vi "Update.vi"(7 "Parent ID":string, 8 "Error In":errorcluster, 10 "Option String":string, 11 "Tree Manager":T1) -> (0 "Error Out":errorcluster, 3 "Tree Manager":T1)   [LabVIEW 2020, in "NI_VIAnCFGDataStructure.lvlib" / "Tree.lvclass"]
doc: "Call the Update method defined for all the Tree Data types stored as the arguments of the specified Tree. If you prefer to call the Update on a specific argument only Get, Update and Set the argument using basic Tree API calls.\n\nTo define new functionality for Update create child classes of Tree Data.lvclass and override the behavior of the parent for Update method."
uses:
  <vilib>/addons/analyzer/VIAnCFGDataStructure/Tree Manager/Tree.lvclass
  <vilib>/addons/analyzer/VIAnCFGDataStructure/Tree Manager/Typedefs/Session Handle.ctl
  <vilib>/addons/analyzer/VIAnCFGDataStructure/Tree Manager/Tree.lvclass/Tree.ctl
  <vilib>/addons/analyzer/VIAnCFGDataStructure/Tree Data/Tree Data.lvclass
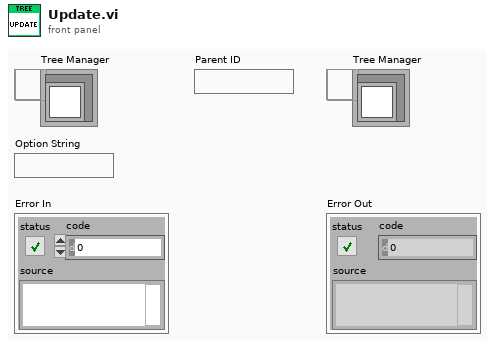
[diagram p1: front panel]
types:
  T1 = typedef "NI_VIAnCFGDataStructure.lvlib/Tree.lvclass/Session Handle.ctl" = refnum<data-value>
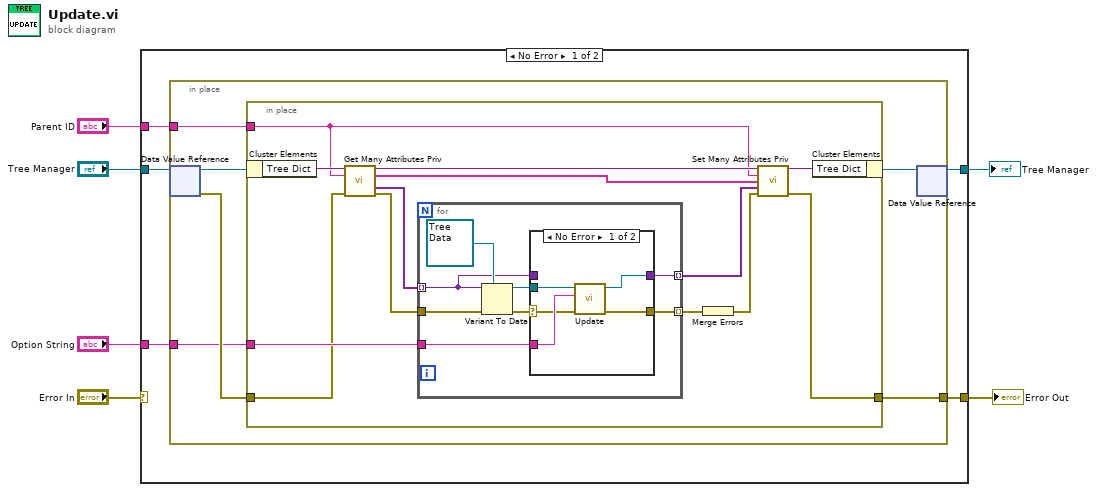
[diagram p0: block diagram]
diagram:
  n1 = case shown="No Error" "Error In" {
    selector: "Error In" -> [_ w45]
    tunnel: "Tree Manager" -> [w11 w46]
    tunnel: [w10 w46] -> w5
    tunnel: [w9 w45] -> w3
    tunnel: "Parent ID" -> [w8 _]
    tunnel: "Option String" -> [w7 _]
    frame No Error {
      n2 = in-place {
        in-place-border: [w16] -> w9
        in-place-border: w8 -> [w13]
        in-place-border: w7 -> [w12]
        n3 = in-place-dvr #1(w11) -> (w17:refnum<class "Tree.lvclass">, w14:errorcluster)
        n4 = in-place {
          in-place-border: [w19] -> w16
          in-place-border: w14 -> [w22]
          in-place-border: w13 -> [w20]
          in-place-border: w12 -> [w26]
          n5 = in-place-cluster #2(w17) -> ("Tree Dict"=w30:variant)
          n6 = call <vilib>:"Get Many Attributes Priv.vi"("Tree Dictionary In"=w30, "Unique ID"=w20, "error in"=w22) -> ("Tree Dictionary Out"=w29:variant, "Attribute Names"=w18:string[], "Attribute Values"=w27:variant[], "error out"=w23:errorcluster)  [unwired: 8 in, 1 out]
          n7 = for {
            tunnel: w27 -> [w33] mode=indexing
            tunnel: w26 -> [w35]
            tunnel: [w34] -> w25 mode=indexing
            tunnel: [w32] -> w24 mode=indexing
            tunnel: w23 -> [w31]
            n8 = Variant To Data(error in=w31, type=refnum<class "Tree Data.lvclass"> refnum ("Tree Data.lvclass"), Variant=w33) -> (data=w36:refnum<class "Tree Data.lvclass">, error out=w37:errorcluster)
            n9 = case shown="No Error" w37 {
              selector: w37 -> [w41 _]
              tunnel: w36 -> [w43 _]
              tunnel: w35 -> [w42 _]
              tunnel: [w40 w44] -> w34
              tunnel: w33 -> [_ w44]
              tunnel: [w39 _] -> w32
              frame No Error {
                n10 = call-dynamic "Update.vi"("Error In"=w41, "Option String"=w42, "Tree Data In"=w43) -> ("Error Out"=w39:errorcluster, "Tree Data Out"=w40:refnum<class "Tree Data.lvclass">)  [unwired: 7 in]
              }
              frame Error {
              }
            }
          }
          n11 = Merge Errors(w24) -> (w21:errorcluster)
          n12 = call <vilib>:"Set Many Attributes Priv.vi"("Tree Dictionary Out"=w29, "Unique ID"=w20, "Name"=w18, "Data"=w25, "error in"=w21) -> ("Tree Dictionary Out"=w28:variant, "error out"=w19:errorcluster)  [unwired: 8 in, 1 out]
          n13 = in-place-cluster #2("Tree Dict"=w28) -> (w15:refnum<class "Tree.lvclass">)
        }
        n14 = in-place-dvr #1(w15) -> (w10:T1)  [unwired: 1 out]
      }
    }
    frame Error {
    }
  }
  "Tree Manager" <- w5
  "Error Out" <- w3
